vi "CreateWindowWithProperties.vi"(8 "No Error":errorcluster, 11 "Properties":T1) -> (0 "Error Out":errorcluster, 3 "Window [SDL_Window *]":i64 format="%.0x")   [LabVIEW 2024, in "SDL3.lvlib" / "Video.lvlib"]
doc: "<B>Summary</B>\nCreate a window with the specified properties.\n\n<B>Remarks</B>\nThese are the supported properties:\n- <B>SDL_PROP_WINDOW_CREATE_ALWAYS_ON_TOP_BOOLEAN</B>: true if the window should be always on top\n- <B>SDL_PROP_WINDOW_CREATE_BORDERLESS_BOOLEAN</B>: true if the window has no window decoration\n- <B>SDL_PROP_WINDOW_CREATE_EXTERNAL_GRAPHICS_CONTEXT_BOOLEAN</B>: true if the window will be used with an externally managed graphics context.\n- <B>SDL_PROP_WINDOW_CREATE_FOCUSABLE_BOOLEAN</B>: true if the window should accept keyboard input (defaults true)\n- <B>SDL_PROP_WINDOW_CREATE_FULLSCREEN_BOOLEAN</B>: true if the window should start in fullscreen mode at desktop resolution\n- <B>SDL_PROP_WINDOW_CREATE_HEIGHT_NUMBER</B>: the height of the window\n- <B>SDL_PROP_WINDOW_CREATE_HIDDEN_BOOLEAN</B>: true if the window should start hidden\n- <B>SDL_PROP_WINDOW_CREATE_HIGH_PIXEL_DENSITY_BOOLEAN</B>: true if the window uses a high pixel density buffer if possible\n- <B>SDL_PROP_WINDOW_CREATE_MAXIMIZED_BOOLEAN</B>: true if the window should start maximized\n- <B>SDL_PROP_WINDOW_CREATE_MENU_BOOLEAN</B>: true if the window is a popup menu\n- <B>SDL_PROP_WINDOW_CREATE_METAL_BOOLEAN</B>: true if the window will be used with Metal rendering\n- <B>SDL_PROP_WINDOW_CREATE_MINIMIZED_BOOLEAN</B>: true if the window should start minimized\n- <B>SDL_PROP_WINDOW_CREATE_MODAL_BOOLEAN</B>: true if the window is modal to its parent\n- <B>SDL_PROP_WINDOW_CREATE_MOUSE_GRABBED_BOOLEAN</B>: true if the window starts with grabbed mouse focus\n- <B>SDL_PROP_WINDOW_CREATE_OPENGL_BOOLEAN</B>: true if the window will be used with OpenGL rendering\n- <B>SDL_PROP_WINDOW_CREATE_PARENT_POINTER</B>: an SDL_Window that will be the parent of this window, required for windows with the \"tooltip\", \"menu\", and \"modal\" properties\n- <B>SDL_PROP_WINDOW_CREATE_RESIZABLE_BOOLEAN</B>: true if the window should be resizable\n- <B>SDL_PROP_WINDOW_CREATE_TITLE_STRING</B>: the title of the window, in UTF-8 encoding\n- <B>SDL_PROP_WINDOW_CREATE_TRANSPARENT_BOOLEAN</B>: true if the window show transparent in the areas with alpha of 0\n- <B>SDL_PROP_WINDOW_CREATE_TOOLTIP_BOOLEAN</B>: true if the window is a tooltip\n- <B>SDL_PROP_WINDOW_CREATE_UTILITY_BOOLEAN</B>: true if the window is a utility window, not showing in the task bar and window list\n- <B>SDL_PROP_WINDOW_CREATE_VULKAN_BOOLEAN</B>: true if the window will be used with Vulkan rendering\n- <B>SDL_PROP_WINDOW_CREATE_WIDTH_NUMBER</B>: the width of the window\n- <B>SDL_PROP_WINDOW_CREATE_X_NUMBER</B>: the x position of the window, or <B>SDL_WINDOWPOS_CENTERED</B>, defaults to <B>SDL_WINDOWPOS_UNDEFINED</B>. This is relative to the parent for windows with the \"tooltip\" or \"menu\" property set.\n- <B>SDL_PROP_WINDOW_CREATE_Y_NUMBER</B>: the y position of the window, or <B>SDL_WINDOWPOS_CENTERED</B>, defaults to <B>SDL_WINDOWPOS_UNDEFINED</B>. This is relative to the parent for windows with the \"tooltip\" or \"menu\" property set.\n\nThese are additional supported properties on macOS:\n- <B>SDL_PROP_WINDOW_CREATE_COCOA_WINDOW_POINTER</B>: the (__unsafe_unretained) NSWindow associated with the window, if you want to wrap an existing window.\n- <B>SDL_PROP_WINDOW_CREATE_COCOA_VIEW_POINTER</B>: the (__unsafe_unretained) NSView associated with the window, defaults to [window contentView]\n\nThese are additional supported properties on Wayland:\n- <B>SDL_PROP_WINDOW_CREATE_WAYLAND_SURFACE_ROLE_CUSTOM_BOOLEAN</B>\ntrue if the application wants to use the Wayland surface for a custom role and does not want it attached to an XDG toplevel window. See README/wayland for more information on using custom surfaces.\n- <B>SDL_PROP_WINDOW_CREATE_WAYLAND_CREATE_EGL_WINDOW_BOOLEAN</B>\ntrue if the application wants an associated wl_egl_window object to be created and attached to the window, even if the window does not have the OpenGL property or <B>SDL_WINDOW_OPENGL</B> flag set.\n- <B>SDL_PROP_WINDOW_CREATE_WAYLAND_WL_SURFACE_POINTER</B>\nthe wl_surface associated with the window, if you want to wrap an existing window. See README/wayland for more information.\n\nThese are additional supported properties on Windows:\n- <B>SDL_PROP_WINDOW_CREATE_WIN32_HWND_POINTER</B>: the HWND associated with the window, if you want to wrap an existing window.\n- <B>SDL_PROP_WINDOW_CREATE_WIN32_PIXEL_FORMAT_HWND_POINTER</B>: optional, another window to share pixel format with, useful for OpenGL windows\n\nThese are additional supported properties with X11:\n- <B>SDL_PROP_WINDOW_CREATE_X11_WINDOW_NUMBER</B>: the X11 Window associated with the window, if you want to wrap an existing window.\n\nThe window is implicitly shown if the \"hidden\" property is not set.\n\nWindows with the \"tooltip\" and \"menu\" properties are popup windows and have the behaviors and guidelines outlined in <B>SDL_CreatePopupWindow()</B>.\n\nIf this window is being created to be used with an SDL_Renderer, you should not add a graphics API specific property (<B>SDL_PROP_WINDOW_CREATE_OPENGL_BOOLEAN</B>, etc), as SDL will handle that internally when it chooses a renderer. However, SDL might need to recreate your window at that point, which may cause the window to appear briefly, and then flicker as it is recreated. The correct approach to this is to create the window with the <B>SDL_PROP_WINDOW_CREATE_HIDDEN_BOOLEAN</B> property set to true, then create the renderer, then show the window with <B>SDL_ShowWindow()</B>."
uses:
  <vilib>/Utility/error.llb/Error Cluster From Error Code.vi
  Video.lvlib
  Error/Error.lvlib
  Lib/SDL3-32.dll
  Properties/PropertiesID--integer.ctl
  Properties/Properties.lvlib
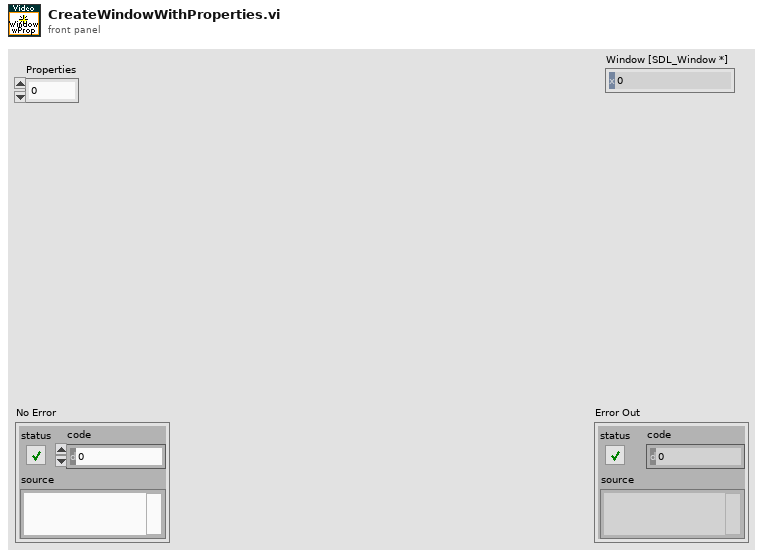
[diagram p1: front panel]
types:
  T1 = typedef "SDL3.lvlib/Properties.lvlib/PropertiesID--integer.ctl" = u32
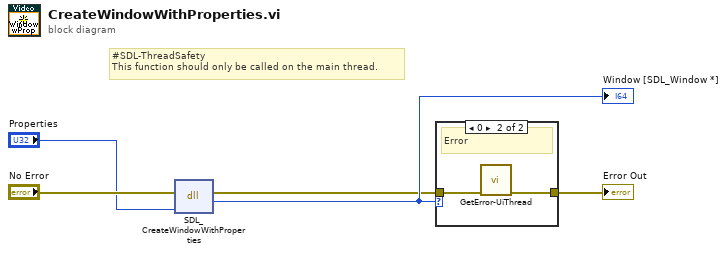
[diagram p0: block diagram]
diagram:
  # "#SDL-ThreadSafety\nThis function should only be called on the main thread."
  n1 = dll-call lib="C:/Users/Thomas/Documents/Projects/LV-SDL3/Lib/SDL3-*.*" fn="SDL_CreateWindowWithProperties"(error in="No Error", "props"="Properties") -> (error out=w2:errorcluster, "return type"=w3:i64)  [unwired: 3 in, 1 out]
  "Window [SDL_Window *]" <- w3
  n2 = case shown="0" w3 {
    tunnel: w2 -> [w6 w8]
    tunnel: [w6 w7] -> w4
    frame Default {
      # "Ok"
    }
    frame 0 {
      # "Error"
      n3 = call "GetError-UiThread.vi"("No Error"=w8) -> ("error out"=w7:errorcluster)  [unwired: 10 in]
    }
  }
  "Error Out" <- w4
